vi "ImportSession.vi"(8 "error in (no error)":errorcluster, 10 "Tuple":T1={"mouse_id"=1217.0, "session_timestamp"="", "pulse_duration"=0.0, "intertrial_interval"=0.0, "file_name"="", "depth"=0.0, "notes"=""}, 11 "Database in":refnum<class "Database.lvclass">) -> (0 "error out":errorcluster, 3 "Database out":refnum<class "Database.lvclass">)   [LabVIEW 2014, in "Database.lvclass"]
uses:
  Database.lvclass
  Database.lvclass/Database.ctl
  <vilib>/addons/database/NI_Database_API.lvlib
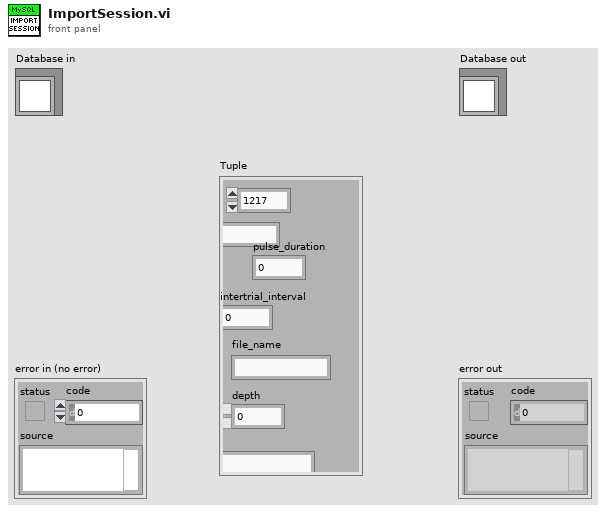
[diagram p1: front panel]
types:
  T1 = cluster{"mouse_id":dbl, "session_timestamp":string, "pulse_duration":dbl, "intertrial_interval":dbl, "file_name":string, "depth":dbl, "notes":string}
  T2 = typedef "NI_Database_API.lvlib/Conn ObjectReference.ctl" = refnum<k1>
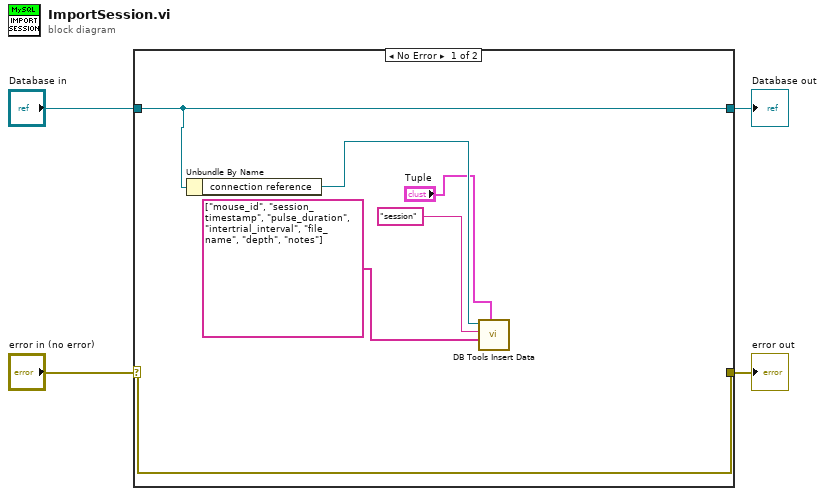
[diagram p0: block diagram]
diagram:
  n1 = case shown="No Error" "error in (no error)" {
    selector: "error in (no error)" -> [w10 w12]
    tunnel: [w10 w12] -> w3
    tunnel: [w7 w11] -> w1
    tunnel: "Database in" -> [w7 w11]
    frame No Error {
      n2 = Unbundle By Name(w7) -> ("connection reference"=w8:T2)
      n3 = call <vilib>:"DB Tools Insert Data.vi"("data"="Tuple", "columns"=string[] ["mouse_id", "session_timestamp", "pulse_duration", "intertrial_interval", "file_name", "depth", "notes"], "table"="session", "connection reference"=w8) -> ()  [unwired: 6 in, 2 out]
    }
    frame Error {
    }
  }
  "error out" <- w3
  "Database out" <- w1
